vi "Write Scaling coefficients.vi"(8 "error in (no error)":errorcluster, 10 "Scaling coefficients":dbl[][](array[numeric]), 11 "Start Stream Result in":refnum<class "Start Stream Result.lvclass">) -> (0 "error out":errorcluster, 3 "Start Stream Result out":refnum<class "Start Stream Result.lvclass">)   [LabVIEW 2019, in "Start Stream Result.lvclass"]
uses:
  Start Stream Result.lvclass
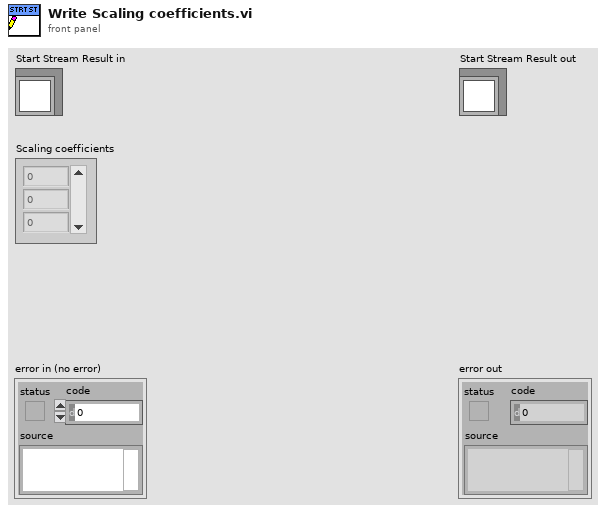
[diagram p1: front panel]
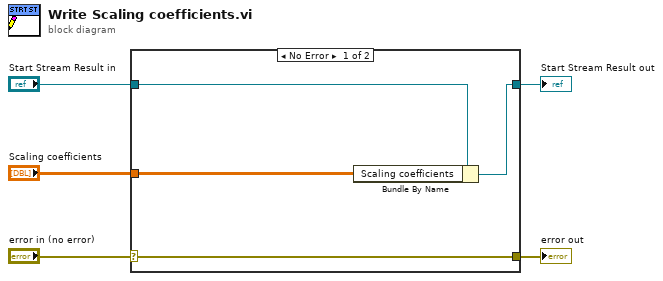
[diagram p0: block diagram]
diagram:
  n1 = case shown="No Error" "error in (no error)" {
    selector: "error in (no error)" -> [w9 w10]
    tunnel: [w9 w10] -> w4
    tunnel: [w7 w11] -> w2
    tunnel: "Start Stream Result in" -> [w8 w11]
    tunnel: "Scaling coefficients" -> [w6 _]
    frame No Error {
      n2 = Bundle By Name(cluster=w8, "Scaling coefficients"=w6) -> (w7:refnum<class "Start Stream Result.lvclass">)
    }
    frame Error {
    }
  }
  "error out" <- w4
  "Start Stream Result out" <- w2
